vi "Tosca-Test Histogram.vi"() -> ()   [LabVIEW 2015]
panel:
  in  "Results":cluster{"name":string, "N":i32[]}[](array[cluster])=[{"name"="Group1", "N"=[1, 2]}, {"name"="Group2", "N"=[1, 1]}, {"name"="Group 3", "N"=[1, 1]}, {"name"="other", "N"=[1]}, {"name"="error", "N"=[1]}]
  out "Histogram":cluster{dbl[], dbl[]}[](graph)=[{[0.625, 1.375], [0.5, 0.5]}, {[1.625, 2.375], [1.0, 1.0]}, {[3.125, 3.875], [0.5, 0.5]}, {[4.125, 4.875], [0.5, 0.5]}, {[5.625, 6.375], [0.5, 0.5]}, {[6.625, 7.375], [0.5, 0.5]}, {[8.125, 8.875], [0.5, 0.5]}, {[9.125, 9.875], [0.5, 0.5]}]
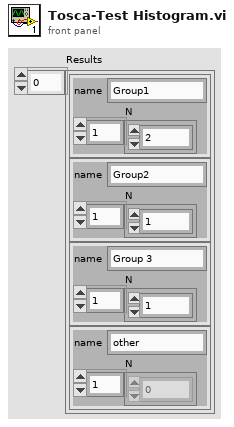
[diagram p1: front panel]
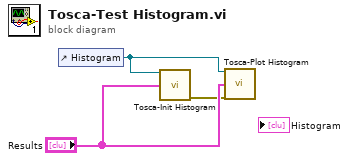
[diagram p0: block diagram]
diagram:
  n1 = control-ref of="Histogram"() -> (w3:refnum<vi>)
  n2 = call "Tosca-Init Histogram.vi"("Histogram"=w3, "Results"="Results") -> ("error out"=w1:errorcluster)  [unwired: 13 in]
  n3 = call "Tosca-Plot Histogram.vi"("Histogram"=w3, "Results"="Results", "error in (no error)"=w1) -> ()  [unwired: 12 in, 1 out]
